vi "OpenFolder.vi"(11 "LabVIEW Data Path":path) -> ()   [LabVIEW 2022 SP3]
uses:
  <vilib>/Platform/browser.llb/Open URL in Default Browser (path).vi
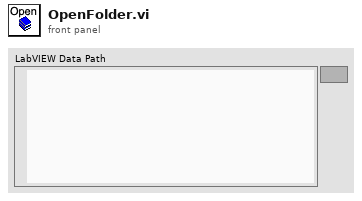
[diagram p1: front panel]
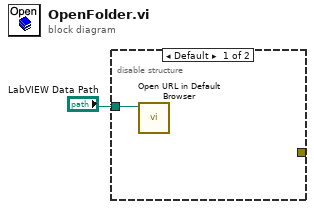
[diagram p0: block diagram]
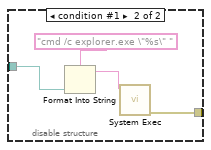
[diagram p2: hidden frame]
diagram:
  n1 = disable-structure shown="Default" {
    disable-tunnel: "LabVIEW Data Path" -> [w2 w5]
    disable-tunnel: [_ w3] -> _
    frame condition #0 (active) {
      n2 = call-poly <vilib>:"Open URL in Default Browser.vi"("path"=w2) -> ()  [unwired: 5 in, 2 out]
    }
    frame condition #1 {
      n3 = Format Into String(format string="cmd /c explorer.exe \"%s\" ", w5) -> (resulting string=w4:string)  [unwired: 2 in, 1 out]
      n4 = call <vilib>:"System Exec.vi"("command line"=w4) -> ("error out"=w3:errorcluster)  [unwired: 7 in, 3 out]
    }
  }
